vi "Set speed.vi"(8 "error in (no error)":errorcluster, 11 "StageSPIM in":refnum<class "StageSPIM.lvclass">) -> (0 "error out":errorcluster, 3 "StageSPIM out":refnum<class "StageSPIM.lvclass">)   [LabVIEW 2012, in "StageSPIM.lvclass"]
uses:
  StageSPIM.lvclass
  StageSPIM.lvclass/StageSPIM.ctl
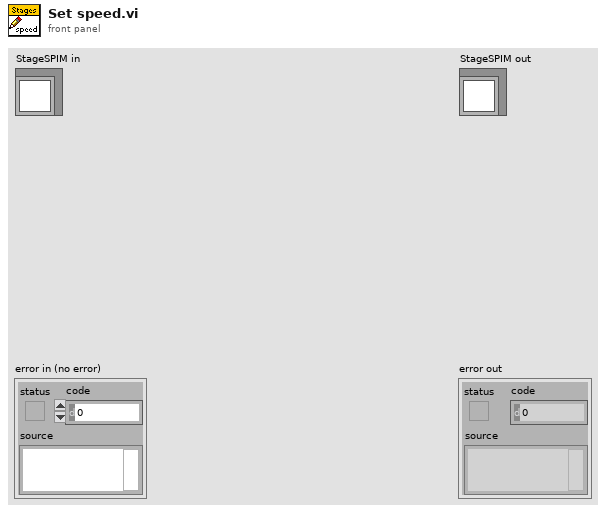
[diagram p1: front panel]
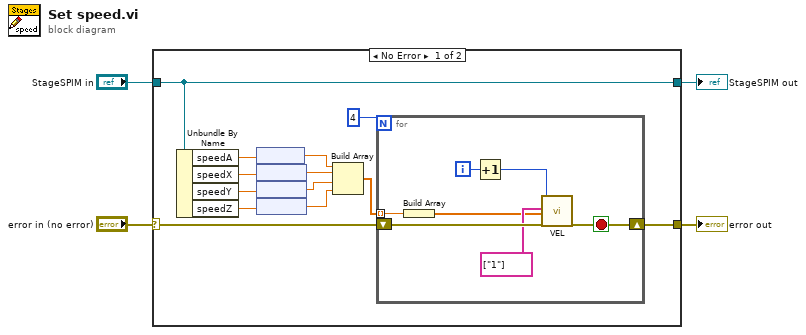
[diagram p0: block diagram]
diagram:
  n1 = case shown="No Error" "error in (no error)" {
    selector: "error in (no error)" -> [w17 w26]
    tunnel: [w16 w26] -> w3
    tunnel: [w14 w25] -> w1
    tunnel: "StageSPIM in" -> [w14 w25]
    frame No Error {
      n2 = Unbundle By Name(w14) -> ("speedA"=w11:dbl[unit], "speedX"=w10:dbl[unit], "speedY"=w13:dbl[unit], "speedZ"=w12:dbl[unit])
      n3 = node(w11) -> (w9:dbl)
      n4 = node(w10) -> (w8:dbl)
      n5 = node(w13) -> (w7:dbl)
      n6 = node(w12) -> (w6:dbl)
      n7 = Build Array(w9, w8, w7, w6) -> (w5:dbl[])
      n8 = for {
        N: 4 -> [_]
        shift-right: [w20] -> w16
        shift-left: w17 -> [w24]
        tunnel: w5 -> [w19] mode=indexing
        i -> [w22]
        stop <- w20 stop-if-true
        n9 = Build Array(w19) -> (w18:dbl[])
        n10 = Increment(x=w22) -> (x+1=w21:i32)
        n11 = call "VEL.vi"("System no."=w21, "Axes to set"=string[] ["1"], "Velocity values"=w18, "error in"=w24) -> ("error out"=w20:errorcluster)  [unwired: 14 in, 1 out]
      }
    }
    frame Error {
    }
  }
  "error out" <- w3
  "StageSPIM out" <- w1
